vi "Average.vi"(9 "B":dbl, 10 "A":dbl) -> (2 "Avg":dbl)   [LabVIEW 2011]
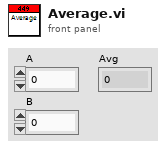
[diagram p1: front panel]
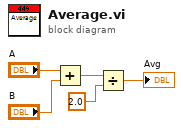
[diagram p0: block diagram]
diagram:
  n1 = Add(x="A", y="B") -> (x+y=w3:dbl)
  n2 = Divide(x=w3, y=2.0) -> (x/y=→"Avg":dbl)
